vi "Parse HTTP Response Headers.vi"(11 "headers":string="HTTP/1.1 200 OK\r\nAccess-Control-Expose-Headers: Content-Length\r\nETag: \"v3a0\"\r\nExpires: Sat, 18 Jan 2020 16:15:15 GMT\r\nContent-Disposition: inline;filename=\"unnamed.jpg\"\r\nContent-Type: image/jpeg\r\nVary: Origin\r\nAccess-Control-Allow-Origin: *\r\nTiming-Allow-Origin: *\r\nX-Content-Type-Options: nosniff\r\nDate: Fri, 17 Jan 2020 20:37:42 GMT\r\nServer: fife\r\nContent-Length: 2537\r\nX-XSS-Protection: 0\r\nAge: 449\r\nCache-Control: public, max-age=86400, no-transform\r\nAlt-Svc: quic=\":443\"; ma=2592000; v=\"46,43\",h3-Q050=\":443\"; ma=2592000,h3-Q049=\":443\"; ma=2592000,h3-Q048=\":443\"; ma=2592000,h3-Q046=\":443\"; ma=2592000,h3-Q043=\":443\"; ma=2592000\r\n\r\n") -> (1 "Response Message":string, 2 "Response Code":i32, 3 "map":map{string, string}(c390))   [LabVIEW 2019, in "Useful HTTP VIs.lvlib"]
uses:
  Useful HTTP VIs/Useful HTTP VIs.lvlib
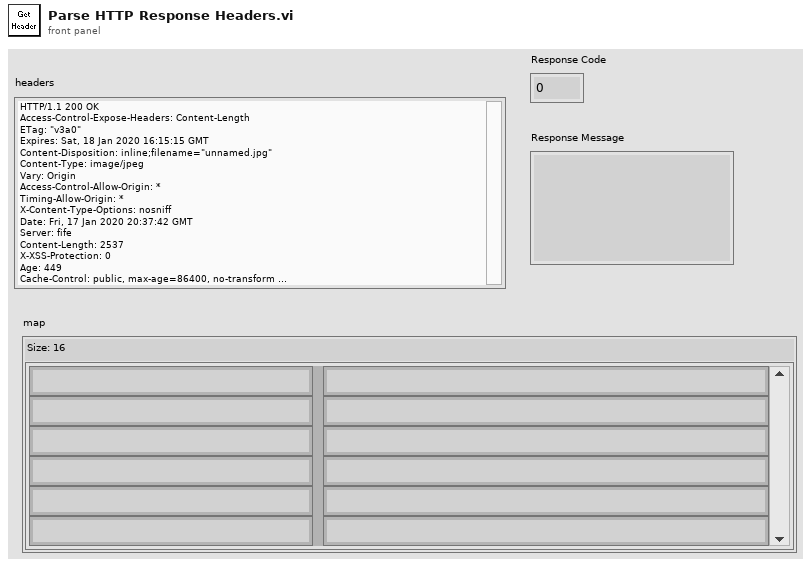
[diagram p1: front panel]
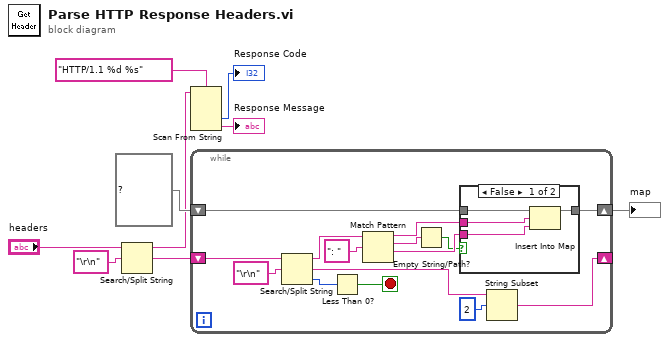
[diagram p0: block diagram]
diagram:
  n1 = Search/Split String(string="headers", search string/char (-)="\r\n") -> (substring before match=w4:string, match + rest of string=w5:string)  [unwired: 1 in, 1 out]
  n2 = Scan From String(format string="HTTP/1.1 %d %s", input string=w4) -> (output 1=→"Response Code":i32, output 2=→"Response Message":string)  [unwired: 4 in, 3 out]
  n3 = while {
    shift-right: [w23] -> w8
    shift-left: map{string, string} {} ("map") -> [w24]
    shift-right: [w10] -> _
    shift-left: w5 -> [w18]
    stop <- w22 stop-if-true
    n4 = Search/Split String(string=w18, search string/char (-)="\r\n") -> (substring before match=w16:string, match + rest of string=w12:string, offset of match=w13:i32)  [unwired: 1 in]
    n5 = Less Than 0?(x=w13) -> (x < 0?=w22:bool)
    n6 = Match Pattern(string=w16, regular expression=": ") -> (before substring=w20:string, match substring=w15:string, after substring=w19:string)  [unwired: 1 in, 1 out]
    n7 = Empty String/Path?(string/path=w15) -> (empty?=w14:bool)
    n8 = case shown="False" w14 {
      tunnel: w24 -> [w28 w29]
      tunnel: [w27 w29] -> w23
      tunnel: w20 -> [w26 _]
      tunnel: w19 -> [w25 _]
      frame False {
        n9 = Insert Into Map(map in=w28, key=w26, value=w25) -> (map out=w27:map{string, string})  [unwired: 2 out]
      }
      frame True {
      }
    }
    n10 = String Subset(string=w12, offset (0)=2) -> (substring=w10:string)  [unwired: 1 in]
  }
  "map" <- w8
